vi "002 DataSaveThread.vi"(8 "Caller":refnum<queue>, 9 "Project":string, 10 "Path":path=path "D:/NBT/Code/NBT-TestPlatform 20230715/Config/NBT/NBT_V3.0.0/Default/DataSave/Save/Save01", 11 "Exit":refnum<user-event>) -> ()   [LabVIEW 2020]
uses:
  Alin/QMH/Queue Message.ctl
  9999 SubVI/000_DataSave/Save Type.ctl
  <vilib>/Utility/file.llb/Read Delimited Spreadsheet (string).vi
  <vilib>/Utility/config.llb/Read Key (String).vi
  <vilib>/Utility/config.llb/NI_LVConfig.lvlib
panel:
  out "Wave":waveform(sgl)(graph)
  out "C1":u64(graph)
  out "C2":T1(graph)
  out "C3":i32(graph)
  out "QS":string
  out "QN":i32
  in  "Stop":bool
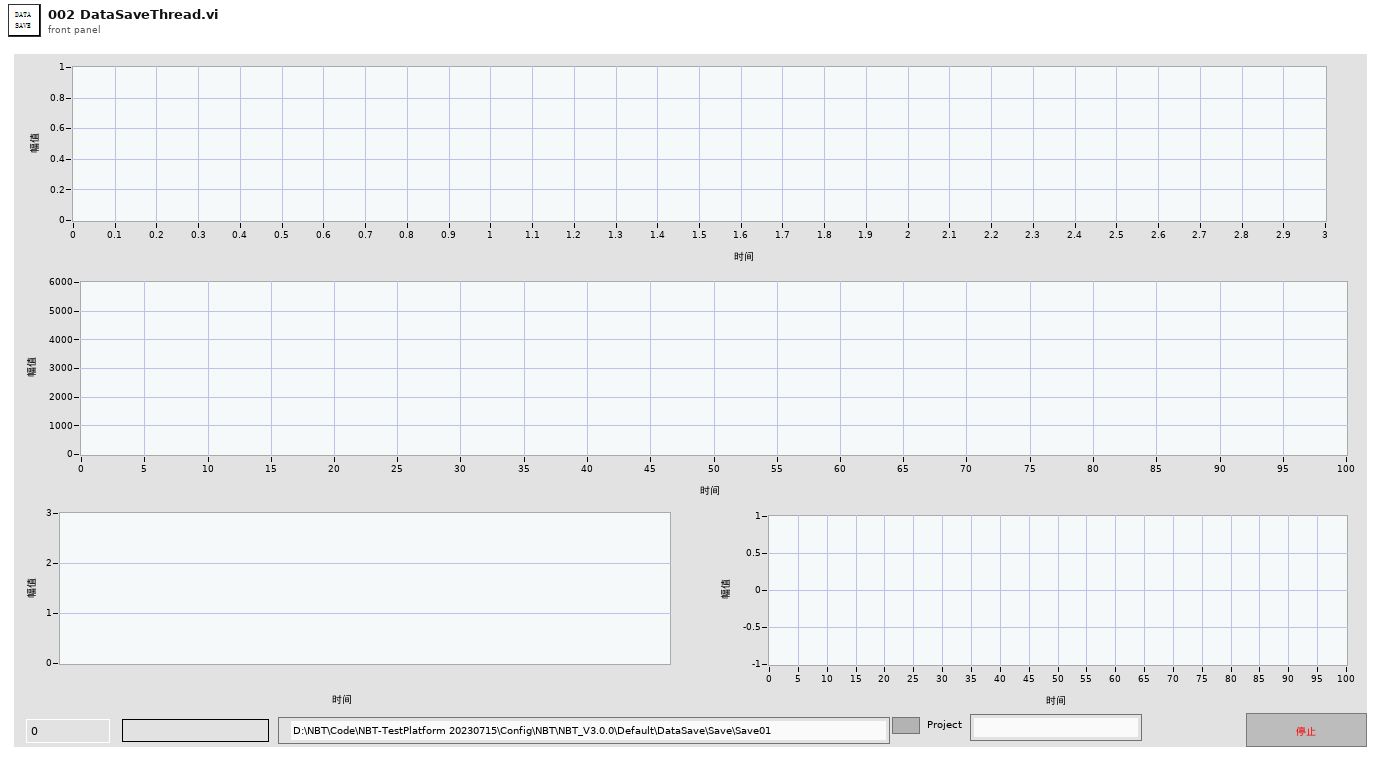
[diagram p1: front panel]
types:
  T1 = cluster{"seconds since 1Jan1904":timestamp, i32}[]
  T2 = typedef "Save Type.ctl" = cluster{"Project":string, "Path":path, "Name":string, "Wave":waveform(sgl)}
  T3 = cluster{"DPath":path, "Last":u64, "Interval":u64, "Max":i32, "File":cluster{"File":string, "Max":i64}, "Wave":map{string, waveform(sgl)}, "Names":string[], "Time":cluster{"UP":u64, "LOW":u64}, "Project":string, "WQ":refnum<queue>, "SQ":map{string, refnum<queue>}, "Save Name":string, "Type":T2, "Caller":refnum<queue>}
  T4 = enum8{"Enabled", "Disabled", "Disabled and Grayed Out"}
  T5 = typedef "NI_LVConfig.lvlib/Config Data RefNum.ctl" = refnum<k1>
  T6 = enum32{"Invalid", "Standard", "Closed", "Hidden", "Minimized", "Maximized"}
  T7 = typedef "SDQ Data Type.ctl" = cluster{"CAN Length":string, "CAN Name":string, "CAN ID":string, "CAN Type":string, "Test Item":string, "Byte Order":string, "Instruction":string, "Control Type":string, "Group":string, "Offset":dbl, "Coefficient":dbl, "Write Enable":bool, "Lable Type":string, "Key?":string, "Set Value":string, "Upper":dbl, "Lower":dbl, "Unit":string, "Formula":string, "Test Item Type":string, "Length":i32, "Address":string, "Name":string, "Identifier":string, "Data Type":string, "Enumerate?":string, "Enumerate List":string, "Data":string, "Source":string}
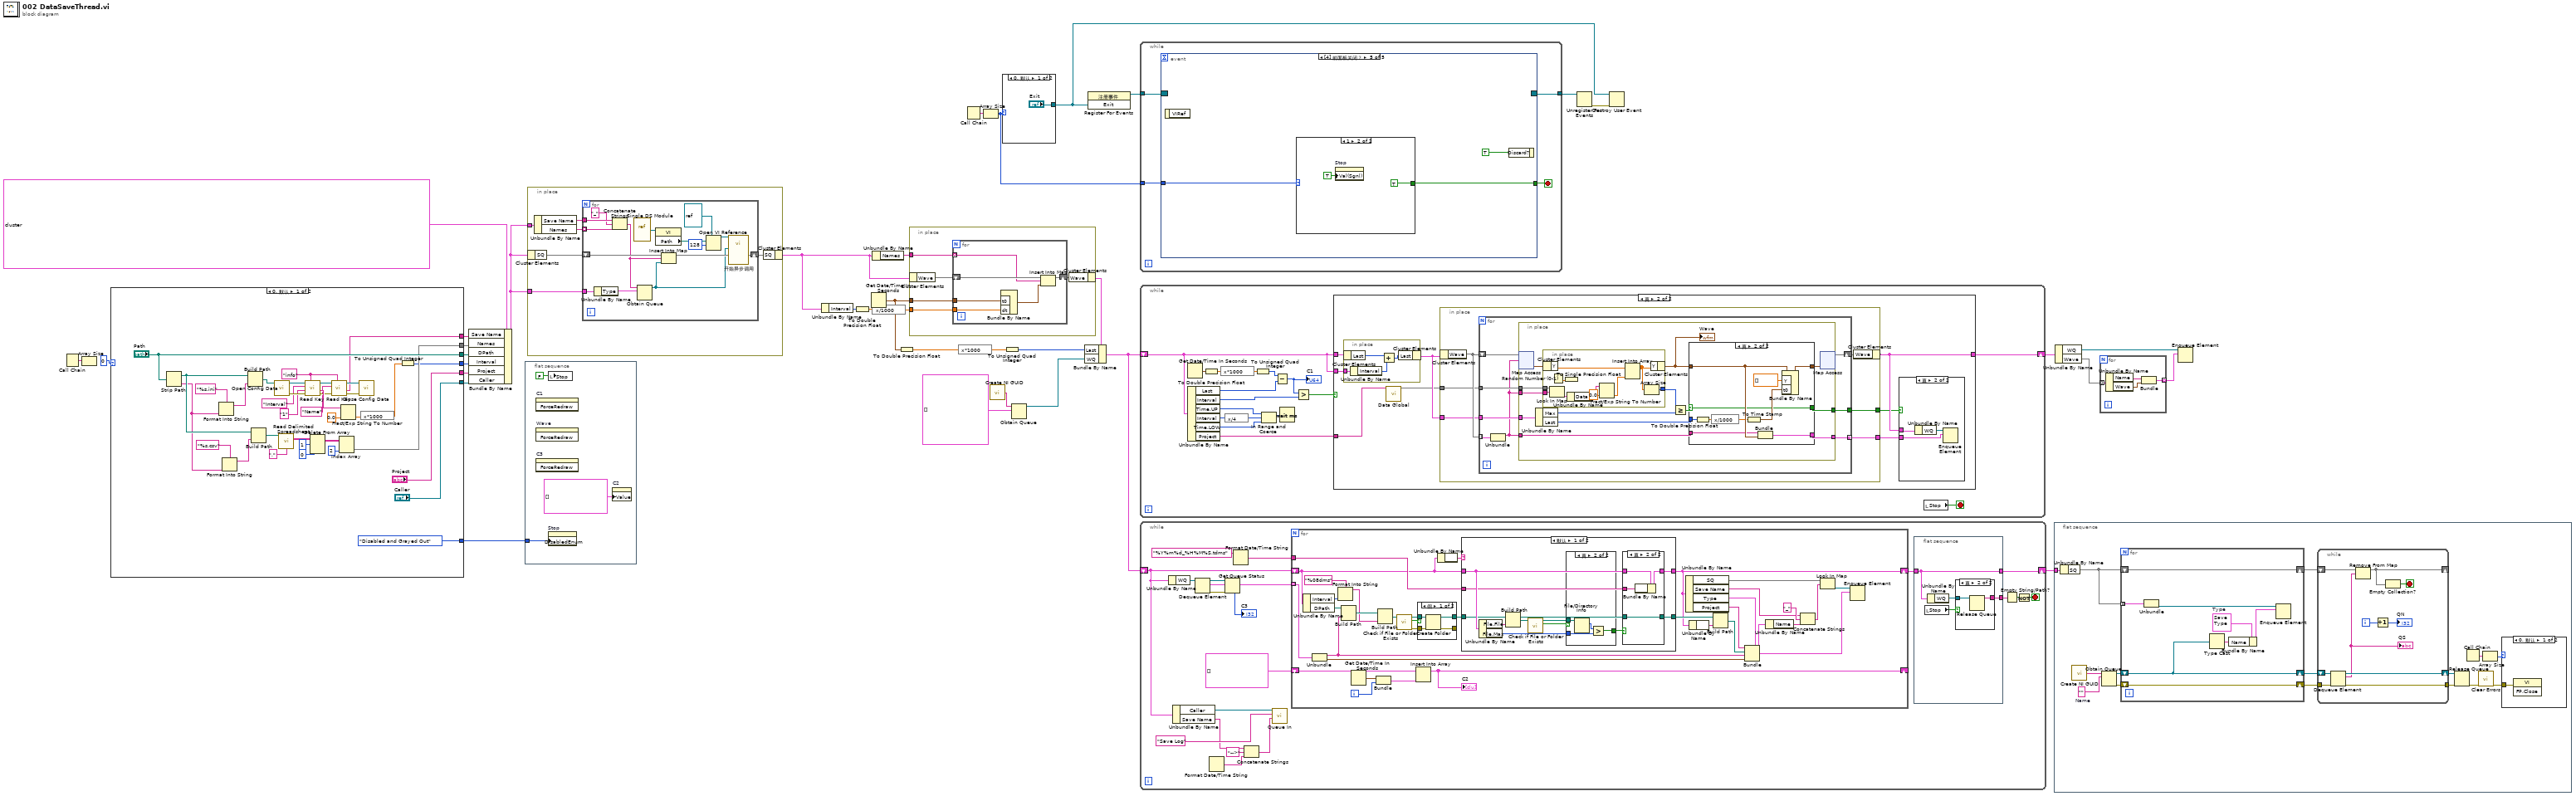
[diagram p0: block diagram]
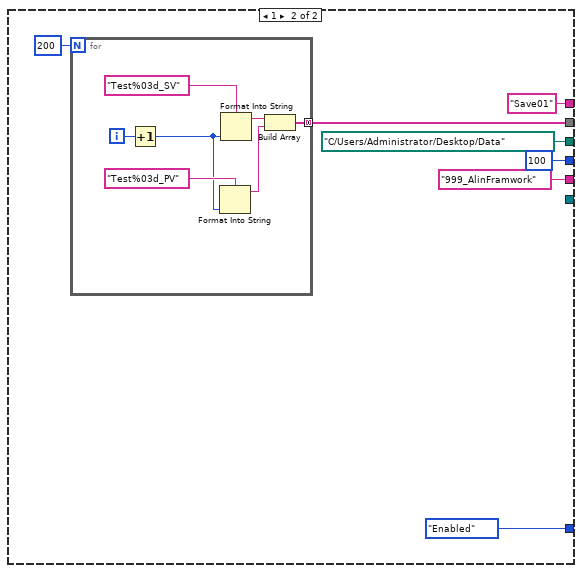
[diagram p2: hidden frame]
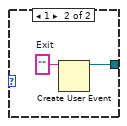
[diagram p3: hidden frame]
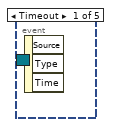
[diagram p5: hidden frame]
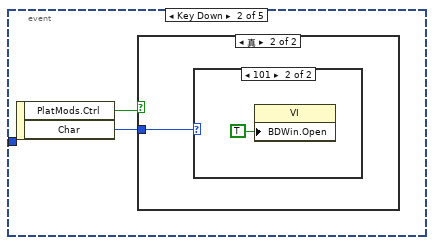
[diagram p6: hidden frame]
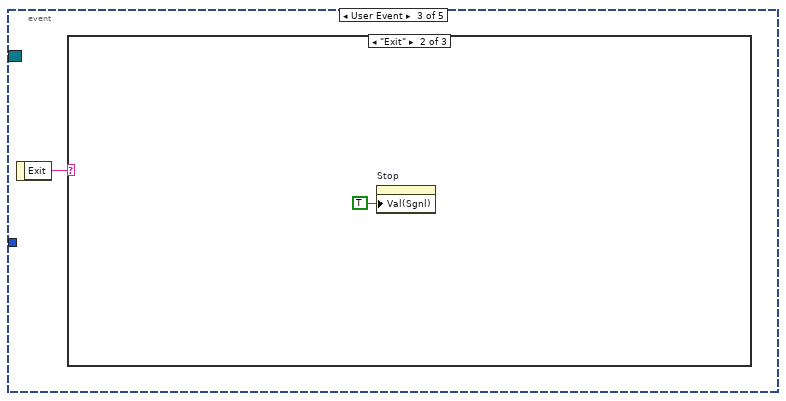
[diagram p9: hidden frame]
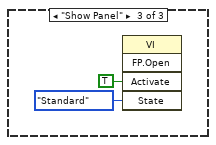
[diagram p11: hidden frame]
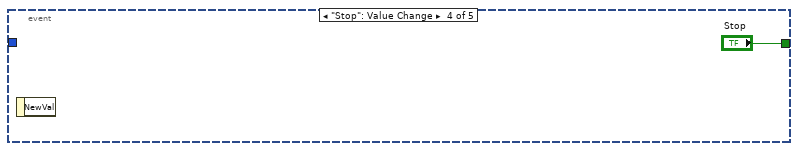
[diagram p12: hidden frame]
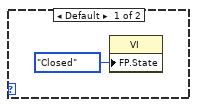
[diagram p13: hidden frame]
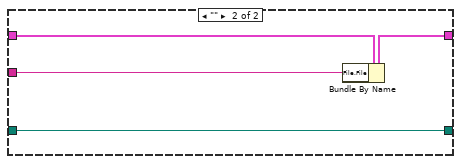
[diagram p17: hidden frame]
diagram:
  n1 = Call Chain() -> (call chain=w11:string[])
  n2 = Array Size(array=w11) -> ()  [unwired: 1 out]
  n3 = case shown="0, 默认" 0 {
    tunnel: ["Path" path "C:/Users/Administrator/Desktop/Data" ("基路径")] -> w26
    tunnel: [w48 u64 100 ("Interval")] -> w25
    tunnel: [w57 w75] -> w23
    tunnel: [T4."Disabled and Grayed Out" ("禁用") T4."Enabled" ("禁用")] -> w9
    tunnel: ["Project" "999_AlinFramwork" ("Project")] -> w8
    tunnel: ["Caller" _] -> w3
    tunnel: [w37 "Save01" ("value")] -> w2
    frame 0, Default {
      w39 = "info" ("section")
      n4 = Strip Path(path="Path") -> (stripped path=w66:path, name=w65:string)
      n5 = Format Into String(format string="%s.ini" ("格式字符串"), w65) -> (resulting string=w69:string)  [unwired: 2 in, 1 out]
      n6 = Format Into String(format string="%s.csv" ("格式字符串"), w65) -> (resulting string=w68:string)  [unwired: 2 in, 1 out]
      n7 = Build Path(base path=w66, name or relative path=w69) -> (appended path=w53:path)
      n8 = Build Path(base path=w66, name or relative path=w68) -> (appended path=w64:path)
      n9 = call <vilib>:"Open Config Data.vi"("configuration file path"=w53) -> ("error out"=w55:errorcluster, "refnum"=w56:T5)  [unwired: 8 in, 1 out]
      n10 = call-poly <vilib>:"Read Delimited Spreadsheet.vi"("file path (dialog if empty)"=w64, "delimiter (\\t)"="," ("delimiter (\\t)")) -> ("all rows"=w62:string[][])  [unwired: 8 in, 5 out]
      n11 = call-poly <vilib>:"Read Key.vi"("section"=w39, "error in (no error)"=w55, "default value"="1", "key"="Interval", "refnum"=w56) -> ("error out"=w42:errorcluster, "value"=w51:string, "refnum out"=w43:T5)  [unwired: 3 in, 1 out]
      n12 = Delete From Array(array=w62, length=1 ("长度"), index (row)=0 ("索引 (行)")) -> (array with subset deleted=w59:string[][])  [unwired: 1 in, 1 out]
      n13 = call-poly <vilib>:"Read Key.vi"("section"=w39, "error in (no error)"=w42, "key"="Name", "refnum"=w43) -> ("error out"=w41:errorcluster, "value"=w37:string, "refnum out"=w40:T5)  [unwired: 4 in, 1 out]
      n14 = Index Array(array=w59, index (col)=2 ("禁用的索引 (列)")) -> (element=w57:string[])  [unwired: 1 in]
      n15 = Fract/Exp String To Number(string=w51, default (0 dbl)=sgl 0.0 ("默认(0 DBL)")) -> (number=w49:sgl)  [unwired: 2 in, 1 out]
      n16 = call <vilib>:"Close Config Data.vi"("error in (no error)"=w41, "refnum"=w40) -> ()  [unwired: 8 in, 2 out]
      n17 = expression code="x*1000"(w49) -> (w47:sgl)
      n18 = To Unsigned Quad Integer(1:w47) -> (0:w48:u64)
    }
    frame 1 {
      n19 = for {
        N: 200 -> [_]
        tunnel: [w80] -> w75 mode=concatenating
        i -> [w83]
        n20 = Increment(x=w83) -> (x+1=w79:i32)
        n21 = Format Into String(format string="Test%03d_PV" ("格式字符串"), w79) -> (resulting string=w81:string)  [unwired: 2 in, 1 out]
        n22 = Format Into String(format string="Test%03d_SV" ("格式字符串"), w79) -> (resulting string=w82:string)  [unwired: 2 in, 1 out]
        n23 = Build Array(w82, w81) -> (w80:string[])
      }
    }
  }
  n24 = Bundle By Name(cluster=T3 {"DPath"=path "", "Last"=0, "Interval"=100, "Max"=100, "File"={"File"="", "Max"=102400}, "Wave"={}, "Names"=[], "Time"={"UP"=500, "LOW"=20}, "Project"="", "WQ"=refnum, "SQ"={}, "Save Name"="Save01", "Type"={"Project"="", "Path"=path "", "Name"="", "Wave"={"t0"=timestamp(0 s since 1904-01-01), "dt"=1.0, "Y"=[]}}, "Caller"=refnum}, "Save Name"=w2, "Names"=w23, "DPath"=w26, "Interval"=w25, "Project"=w8, "Caller"=w3) -> (w18:T3)
  n25 = flat-sequence {
    tunnel: w9 -> [w86]
    frame #0 {
      n26 = invoke on="C1" class="WFChart (严格)" method="ForceRedraw"() -> ()  [unwired: 3 in, 3 out]
      n27 = invoke on="Wave" class="WFGraph (严格)" method="ForceRedraw"() -> ()  [unwired: 3 in, 3 out]
      n28 = invoke on="C3" class="WFChart (严格)" method="ForceRedraw"() -> ()  [unwired: 3 in, 3 out]
      n29 = property on="Stop" class="Bool (严格)"("DisabledEnum"=w86) -> ()  [unwired: 2 in, 2 out]
      n30 = local write "Stop"(FALSE ("Stop")) -> ()
      n31 = property on="C2" class="XYGraph (严格)"("Value"=T1 [] ("C2")) -> ()  [unwired: 2 in, 2 out]
    }
  }
  n32 = in-place {
    in-place-border: w18 -> [w94]
    in-place-border: w18 -> [w89]
    n33 = in-place-cluster #1(w18) -> ("SQ"=w92:map{string, refnum<queue>})
    n34 = Unbundle By Name(w94) -> ("Save Name"=w90:string, "Names"=w93:string[])
    n35 = for {
      tunnel: w93 -> [w106] mode=indexing
      shift-right: [w101] -> w91
      shift-left: w92 -> [w105]
      tunnel: w90 -> [w108]
      tunnel: w89 -> [w103]
      n36 = Unbundle By Name(w103) -> ("Type"=w102:T2)
      n37 = Concatenate Strings(w108, "_" ("字符串"), w106) -> (w104:string)
      n38 = vi-ref "Single DS Module.vi"() -> (w100:refnum<vi>)
      n39 = Obtain Queue(name (unnamed)=w104, element data type=w102) -> (queue out=w95:refnum<queue>)  [unwired: 3 in, 2 out]
      n40 = property class="VI"(reference=w100) -> ("Path"=w99:path)  [unwired: 1 in, 2 out]
      n41 = Insert Into Map(map in=w105, key=w104, value=w95) -> (map out=w101:map{string, refnum<queue>})  [unwired: 2 out]
      n42 = Open VI Reference(type specifier VI Refnum (for type only)=refnum<vi> refnum ("类型说明符VI引用句柄（仅用于类型）"), vi path=w99, options=128 ("选项")) -> (vi reference=w98:refnum<vi>)  [unwired: 3 in, 1 out]
      n43 = call-by-ref "开始异步调用"(reference=w98, "Queue"=w95) -> ()  [unwired: 11 in, 3 out]
    }
    n44 = in-place-cluster #1("SQ"=w91) -> (w7:T3)
  }
  n45 = Unbundle By Name(w7) -> ("Interval"=w6:u64)
  n46 = To Double Precision Float(number=w6) -> (double precision float=w5:dbl)
  n47 = Get Date/Time In Seconds() -> (seconds since 1Jan1904=w33:timestamp)
  n48 = Unbundle By Name(w7) -> ("Names"=w29:string[])
  n49 = expression code="x/1000"(w5) -> (w4:dbl)
  n50 = To Double Precision Float(number=w33) -> (double precision float=w35:dbl)
  n51 = in-place {
    in-place-border: w33 -> [w113]
    in-place-border: w29 -> [w112]
    in-place-border: w4 -> [w109]
    n52 = in-place-cluster #2(w7) -> ("Wave"=w111:map{string, waveform(sgl)})
    n53 = for {
      tunnel: w113 -> [w119]
      tunnel: w109 -> [w118]
      tunnel: w112 -> [w114] mode=indexing
      shift-right: [w116] -> w110
      shift-left: w111 -> [w117]
      n54 = Bundle By Name("t0"=w119, "dt"=w118) -> (w115:waveform(dbl))  [unwired: 1 in]
      n55 = Insert Into Map(map in=w117, key=w114, value=w115) -> (map out=w116:map{string, waveform(sgl)})  [unwired: 2 out]
    }
    n56 = in-place-cluster #2("Wave"=w110) -> (w36:T3)
  }
  n57 = expression code="x*1000"(w35) -> (w34:dbl)
  n58 = Call Chain() -> (call chain=w12:string[])
  n59 = Array Size(array=w12) -> (size(s)=w1:i32)
  n60 = call <vilib>:"Create NI GUID.vi"() -> ("NI GUID"=w27:string)
  n61 = case shown="0, 默认" w1 {
    tunnel: ["Exit" w121] -> w13
    frame 0, Default {
    }
    frame 1 {
      w122 = ""  # Exit
      n62 = Create User Event(user event datatype=w122) -> (user event=w121:refnum<user-event>)  [unwired: 1 in, 1 out]
    }
  }
  n63 = To Unsigned Quad Integer(1:w34) -> (0:w32:u64)
  n64 = Obtain Queue(name (unnamed)=w27, element data type=cluster{"Name":string, "Wave":waveform(sgl)}[] [] ("输出簇")) -> (queue out=w24:refnum<queue>)  [unwired: 3 in, 2 out]
  n65 = Bundle By Name(cluster=w36, "Last"=w32, "WQ"=w24) -> (w31:T3)
  n66 = register-events(w13) -> (reference out=w16:refnum<event-registration>)  [unwired: 2 in, 1 out]
  n67 = while {
    tunnel: w16 -> [w125]
    tunnel: [w124] -> w15
    tunnel: w1 -> [w123]
    stop <- w126 stop-if-true
    n68 = event shown="[4] 前面板关闭？" {
      selector: w125 -> [_ _ _ _ _]
      dyn-events: [_ _ _ _ _] -> w124
      timeout: _ -> [_ _ _ _ _]
      tunnel: [_ _ _ "Stop" w136] -> w126
      tunnel: w123 -> [_ _ _ _ w137]
      event Timeout {
        n69 = event-data() -> ()  [unwired: 1 in, 3 out]
      }
      event Key Down {
        n70 = event-data() -> ("PlatMods.Ctrl"=w128:bool, "Char"=w127:i16)  [unwired: 1 in]
        n71 = case shown="真" w128 {
          tunnel: w127 -> [_ w129]
          frame False {
          }
          frame True {
            n72 = case shown="101" w129 {
              frame 0, Default {
              }
              frame 101 {
                n73 = property class="VI"("BDWin.Open"=TRUE ("程序框图窗口:打开")) -> ()  [unwired: 2 in, 2 out]
              }
            }
          }
        }
      }
      event User Event {
        n74 = event-data() -> ("Exit"=w131:string)  [unwired: 1 in]
        n75 = case shown="\"Exit\"" w131 {
          frame "假", Default {
          }
          frame "Exit" {
            n76 = property on="Stop" class="Bool (严格)"("Val(Sgnl)"=TRUE ("值(信号)")) -> ()  [unwired: 2 in, 2 out]
          }
          frame "Show Panel" {
            n77 = invoke class="VI" method="FP.Open"("Activate"=TRUE ("激活？"), "State"=T6."Standard" ("状态")) -> ()  [unwired: 3 in, 5 out]
          }
        }
      }
      event "Stop": Value Change {
        n78 = event-data() -> ()  [unwired: 1 in, 1 out]
      }
      event Panel Close? {
        n79 = event-data() -> ()  [unwired: 1 in, 1 out]
        n80 = case shown="1" w137 {
          tunnel: [_ TRUE] -> w136
          frame Default {
            n81 = property class="VI"("FP.State"=T6."Closed" ("前面板窗口:状态")) -> ()  [unwired: 2 in, 2 out]
          }
          frame 1 {
            n82 = property on="Stop" class="Bool (严格)"("Val(Sgnl)"=TRUE ("值(信号)")) -> ()  [unwired: 2 in, 2 out]
          }
        }
        n83 = event-data("Discard?"=TRUE ("放弃？")) -> ()  [unwired: 1 in, 1 out]
      }
    }
  }
  n84 = while {
    shift-right: [w153] -> w21
    shift-left: w31 -> [w143]
    stop <- w144 stop-if-true
    n85 = Get Date/Time In Seconds() -> (seconds since 1Jan1904=w158:timestamp)
    n86 = Unbundle By Name(w143) -> ("Last"=w152:u64, "Interval"=w150:u64, "Time.UP"=w147:u64, "Interval"=w146:u64, "Time.LOW"=w145:u64, "Project"=w142:string)
    n87 = To Double Precision Float(number=w158) -> (double precision float=w157:dbl)
    n88 = expression code="x*1000"(w157) -> (w156:dbl)
    n89 = expression code="x/4"(w146) -> (w149:u64)
    n90 = To Unsigned Quad Integer(1:w156) -> (0:w155:u64)
    n91 = In Range and Coerce(upper limit=w147, x=w149, lower limit=w145) -> (coerced(x)=w148:u64)  [unwired: 1 out]
    n92 = Subtract(x=w155, y=w152) -> (x-y=w151:u64)
    "C1" <- w151
    n93 = Wait (ms)(milliseconds to wait=w148) -> ()  [unwired: 1 out]
    n94 = Greater?(x=w151, y=w150) -> (0:w154:bool)
    n95 = case shown="真" w154 {
      tunnel: w143 -> [w159 w167]
      tunnel: [w159 w165] -> w153
      tunnel: w143 -> [_ w162]
      tunnel: w142 -> [_ w161]
      frame False {
      }
      frame True {
        n96 = in-place {
          in-place-border: w162 -> [w173]
          n97 = in-place-cluster #3(w167) -> ("Last"=w174:u64)
          n98 = Unbundle By Name(w173) -> ("Interval"=w172:u64)
          n99 = Add(x=w174, y=w172) -> (x+y=w171:u64)
          n100 = in-place-cluster #3("Last"=w171) -> (w166:T3)
        }
        n101 = call "Data Global.vi"("Name"=w161) -> ("Data Out"=w160:map{string, T7})  [unwired: 7 in, 3 out]
        n102 = in-place {
          in-place-border: w166 -> [w178]
          in-place-border: [w177] -> w164
          in-place-border: [w176] -> w163
          in-place-border: w160 -> [w175]
          n103 = in-place-cluster #4(w166) -> ("Wave"=w180:map{string, waveform(sgl)})
          n104 = for {
            tunnel: w180 -> [w188] mode=indexing
            shift-right: [w186] -> w179
            shift-left: w180 -> [w187]
            tunnel: w178 -> [w185]
            tunnel: [w184] -> w177 mode=indexing
            tunnel: [w183] -> w176
            tunnel: w175 -> [w182]
            n105 = Unbundle(w188) -> ("Name"=w181:string)  [unwired: 1 out]
            n106 = in-place {
              in-place-border: w181 -> [w196]
              in-place-border: w185 -> [w193]
              in-place-border: [w192] -> w184
              in-place-border: [w191] -> w183
              in-place-border: w182 -> [w190]
              in-place-border: w181 -> [w189]
              n107 = in-place-map #5(w187, w181) -> (w197:waveform(sgl))  [unwired: 1 in, 1 out]
              n108 = Unbundle By Name(w193) -> ("Max"=w200:i32, "Last"=w194:u64)
              n109 = in-place {
                in-place-border: [w221] -> w201
                in-place-border: w190 -> [w218]
                in-place-border: w189 -> [w213]
                n110 = in-place-cluster #6(w197) -> ("Y"=w222:sgl[])
                n111 = Look In Map(map=w218, key=w213) -> (value=w217:T7)  [unwired: 1 in, 1 out]
                n112 = Random Number (0-1)() -> (number: 0 to 1=w219:dbl)
                n113 = To Single Precision Float(number=w219) -> ()  [unwired: 1 out]
                n114 = Unbundle By Name(w217) -> ("Data"=w216:string)
                n115 = Fract/Exp String To Number(string=w216, default (0 dbl)=sgl 0.0 ("默认(0 DBL)")) -> (number=w215:sgl)  [unwired: 2 in, 1 out]
                n116 = Insert Into Array(array=w222, new element=w215) -> (w220:sgl[])  [unwired: 1 in]
                n117 = Array Size(array=w220) -> (size(s)=w221:i32)
                n118 = in-place-cluster #6("Y"=w220) -> (w198:waveform(sgl))
              }
              "Wave" <- w198
              n119 = Greater Or Equal?(x=w201, y=w200) -> (x >= y?=w199:bool)
              n120 = case shown="真" w199 {
                selector: w199 -> [_ w203]
                tunnel: w198 -> [w202 w210]
                tunnel: [w202 w211] -> w195
                tunnel: w194 -> [_ w209]
                tunnel: w196 -> [_ w205]
                tunnel: [_ w204] -> w192
                tunnel: [_ w203] -> w191
                frame False {
                }
                frame True {
                  n121 = To Double Precision Float(number=w209) -> (double precision float=w208:dbl)
                  n122 = expression code="x/1000"(w208) -> (w207:dbl)
                  n123 = To Time Stamp(1:w207) -> (0:w206:timestamp)
                  n124 = Bundle("Name"=w205, "Wave"=w210) -> (w204:cluster{"Name":string, "Wave":waveform(sgl)})  [unwired: 1 in]
                  n125 = Bundle By Name(cluster=w210, "Y"=sgl[] [], "t0"=w206) -> (w211:waveform(sgl))
                }
              }
              n126 = in-place-map #5(w195) -> (w186:map{string, waveform(sgl)})  [unwired: 1 in, 2 out]
            }
          }
          n127 = in-place-cluster #4("Wave"=w179) -> (w165:T3)
        }
        n128 = case shown="真" w163 {
          tunnel: w165 -> [_ w170]
          tunnel: w164 -> [_ w168]
          frame False {
          }
          frame True {
            n129 = Unbundle By Name(w170) -> ("WQ"=w169:refnum<queue>)
            n130 = Enqueue Element(queue=w169, element=w168) -> ()  [unwired: 2 in, 3 out]
          }
        }
      }
    }
    n131 = local read "Stop"() -> (w144:bool)
  }
  n132 = while {
    shift-right: [w234] -> w17
    shift-left: w31 -> [w229]
    stop <- w237 stop-if-true
    n133 = Unbundle By Name(w229) -> ("WQ"=w241:refnum<queue>)
    n134 = Unbundle By Name(w229) -> ("Caller"=w228:refnum<queue>, "Save Name"=w226:string)
    n135 = Dequeue Element(queue=w241) -> (queue out=w232:refnum<queue>, element=w242:cluster{"Name":string, "Wave":waveform(sgl)}[], error out=w231:errorcluster)  [unwired: 2 in, 1 out]
    n136 = Format Date/Time String() -> (date/time string=w224:string)  [unwired: 3 in]
    n137 = Get Queue Status(queue=w232, error in (no error)=w231) -> (# elements in queue=→"C3":i32)  [unwired: 1 in, 7 out]
    n138 = Format Date/Time String(time format string (%c)="%Y%m%d_%H%M%S.tdms" ("时间格式字符串(%c)")) -> (date/time string=w239:string)  [unwired: 2 in]
    n139 = Concatenate Strings(w226, "-->" ("字符串"), w224) -> (w223:string)
    n140 = call "Queue In.vi"("Data"=w223, "Message"="Save Log", "Queue In"=w228) -> ()  [unwired: 7 in, 2 out]
    n141 = for {
      tunnel: w242 -> [w282] mode=indexing
      shift-right: [w269] -> w235
      shift-left: w229 -> [w251]
      tunnel: w239 -> [w270]
      shift-right: [w260] -> _
      shift-left: T1 [] ("输出簇") -> [w262]
      i -> [w263]
      n142 = Unbundle By Name(w251) -> ("Interval"=w250:u64, "DPath"=w249:path)
      n143 = Unbundle(w282) -> ("Name"=w266:string, "Wave"=w265:waveform(sgl))
      n144 = Format Into String(format string="%08dms" ("格式字符串"), w250) -> (resulting string=w275:string)  [unwired: 2 in, 1 out]
      n145 = Build Path(base path=w249, name or relative path=w266) -> (appended path=w277:path)
      n146 = Get Date/Time In Seconds() -> (seconds since 1Jan1904=w264:timestamp)
      n147 = Bundle("seconds since 1Jan1904"=w264, w263) -> (w261:cluster{"seconds since 1Jan1904":timestamp, i32})  [unwired: 1 in]
      n148 = Build Path(base path=w277, name or relative path=w275) -> (appended path=w276:path)
      n149 = call <vilib>:"Check if File or Folder Exists.vi"("path"=w276) -> ("error out"=w281:errorcluster, "file or folder exists?"=w279:bool, "dup path"=w280:path)  [unwired: 8 in]
      n150 = Insert Into Array(array=w262, new element=w261) -> (w260:T1)  [unwired: 1 in]
      "C2" <- w260
      n151 = case shown="假" w279 {
        tunnel: w280 -> [w311 w313]
        tunnel: w281 -> [w310 w312]
        tunnel: [w309 w313] -> w273
        tunnel: [w308 w312] -> _
        frame False {
          n152 = Create Folder(path (use dialog)=w311, error in=w310) -> (created path=w309:path, error out=w308:errorcluster)  [unwired: 1 in, 1 out]
        }
        frame True {
        }
      }
      n153 = Unbundle By Name(w251) -> ("File.File"=w274:string)
      n154 = case shown="默认" w274 {
        tunnel: w270 -> [w284 w306]
        tunnel: w273 -> [w288 w304]
        tunnel: w251 -> [w290 w307]
        tunnel: [w289 w305] -> w269
        tunnel: [w287 w304] -> w272
        frame Default {
          n155 = Unbundle By Name(w290) -> ("File.File"=w293:string, "File.Max"=w292:i64)
          n156 = Build Path(base path=w288, name or relative path=w293) -> (appended path=w286:path)
          n157 = call <vilib>:"Check if File or Folder Exists.vi"("path"=w286) -> ("file or folder exists?"=w283:bool, "dup path"=w285:path)  [unwired: 8 in, 1 out]
          n158 = case shown="真" w283 {
            tunnel: w292 -> [_ w296]
            tunnel: [_ w295] -> w291
            tunnel: w285 -> [_ w294]
            frame False {
            }
            frame True {
              n159 = File/Directory Info(path=w294) -> (size=w297:i64)  [unwired: 1 in, 6 out]
              n160 = Greater?(x=w297, y=w296) -> (0:w295:bool)
            }
          }
          n161 = case shown="真" w291 {
            tunnel: w284 -> [_ w301]
            tunnel: w290 -> [w299 w303]
            tunnel: [w299 w302] -> w289
            tunnel: w288 -> [w298 w300]
            tunnel: [w298 w300] -> w287
            frame False {
            }
            frame True {
              n162 = Bundle By Name(cluster=w303, "File.File"=w301) -> (w302:T3)
            }
          }
        }
        frame "" {
          n163 = Bundle By Name(cluster=w307, "File.File"=w306) -> (w305:T3)
        }
      }
      n164 = Unbundle By Name(w269) -> ("SQ"=w255:map{string, refnum<queue>}, "Save Name"=w257:string, "Type"=w259:T2, "Project"=w268:string)
      n165 = Unbundle By Name(w269) -> ("File.File"=w271:string)
      n166 = Build Path(base path=w272, name or relative path=w271) -> (appended path=w267:path)
      n167 = Bundle(cluster=w259, "Project"=w268, "Path"=w267, "Name"=w266, "Wave"=w265) -> (w252:T2)
      n168 = Unbundle By Name(w252) -> ("Name"=w256:string)
      n169 = Concatenate Strings(w257, "_" ("字符串"), w256) -> (w254:string)
      n170 = Look In Map(map=w255, key=w254) -> (value=w253:refnum<queue>)  [unwired: 1 in, 1 out]
      n171 = Enqueue Element(queue=w253, element=w252) -> ()  [unwired: 2 in, 3 out]
    }
    n172 = flat-sequence {
      tunnel: [w245] -> w238
      tunnel: w235 -> [w243]
      tunnel: [w243] -> w234
      frame #0 {
        n173 = local read "Stop"() -> (w246:bool)
        n174 = Unbundle By Name(w243) -> ("WQ"=w244:refnum<queue>)
        n175 = case shown="真" w246 {
          tunnel: w244 -> [_ w248]
          tunnel: [_ w247] -> w245
          frame False {
          }
          frame True {
            n176 = Release Queue(queue=w248) -> (queue name=w247:string)  [unwired: 2 in, 2 out]
          }
        }
      }
    }
    n177 = Empty String/Path?(string/path=w238) -> (empty?=w236:bool)
    n178 = Not(x=w236) -> (.not. x?=w237:bool)
  }
  n179 = Unregister For Events(event registration refnum=w15) -> (error out=w14:errorcluster)  [unwired: 1 in]
  n180 = Destroy User Event(user event=w13, error in=w14) -> ()  [unwired: 1 out]
  n181 = flat-sequence {
    tunnel: w17 -> [w328]
    frame #0 {
      w326 = ""  # Name
      n182 = Unbundle By Name(w328) -> ("SQ"=w324:map{string, refnum<queue>})
      n183 = call <vilib>:"Create NI GUID.vi"() -> ("NI GUID"=w327:string)
      n184 = Obtain Queue(name (unnamed)=w327, element data type=w326) -> (queue out=w325:refnum<queue>, error out=w319:errorcluster)  [unwired: 3 in, 1 out]
      n185 = for {
        tunnel: w324 -> [w347] mode=indexing
        shift-right: [w342] -> w322
        shift-left: w325 -> [w342]
        shift-right: [w341] -> w323
        shift-left: w324 -> [w341]
        shift-right: [w340] -> w318
        shift-left: w319 -> [w340]
        w345 = T2 {"Project"="Exit", "Path"=path "", "Name"="", "Wave"={"t0"=timestamp(0 s since 1904-01-01), "dt"=1.0, "Y"=[]}}  # Type
        n186 = Unbundle(w347) -> ("DQ"=w346:refnum<queue>)  [unwired: 1 out]
        n187 = Type Cast(x=w342) -> (*(type *) &x=w343:string)  [unwired: 1 in]
        n188 = Bundle By Name(cluster=w345, "Name"=w343) -> (w344:T2)
        n189 = Enqueue Element(queue=w346, element=w344) -> ()  [unwired: 2 in, 3 out]
      }
      n190 = while {
        shift-right: [w337] -> _
        shift-left: w323 -> [w338]
        shift-right: [w335] -> w321
        shift-left: w322 -> [w339]
        tunnel: [w334] -> w320
        tunnel: w318 -> [w333]
        i -> [w332]
        stop <- w336 stop-if-true
        n191 = Dequeue Element(queue=w339, error in (no error)=w333) -> (queue out=w335:refnum<queue>, element=w331:string, error out=w334:errorcluster)  [unwired: 1 in, 1 out]
        "QS" <- w331
        n192 = Remove From Map(10:w331, 11:w338) -> (3:w337:map{string, refnum<queue>})  [unwired: 2 out]
        n193 = Increment(x=w332) -> (x+1=→"QN":i32)
        n194 = Empty Collection?(1:w337) -> (0:w336:bool)
      }
      n195 = Release Queue(queue=w321, error in (no error)=w320) -> (error out=w315:errorcluster)  [unwired: 1 in, 2 out]
      n196 = Call Chain() -> (call chain=w317:string[])
      n197 = call <vilib>:"Clear Errors.vi"("error in (no error)"=w315) -> ("error out"=w314:errorcluster)  [unwired: 5 in, 1 out]
      n198 = Array Size(array=w317) -> (size(s)=w316:i32)
      n199 = case shown="0, 默认" w316 {
        tunnel: w314 -> [w329 _]
        frame 0, Default {
          n200 = invoke class="VI" method="FP.Close"(error in=w329) -> ()  [unwired: 2 in, 3 out]
        }
        frame 1 {
        }
      }
    }
  }
  n201 = Unbundle By Name(w21) -> ("WQ"=w22:refnum<queue>, "Wave"=w20:map{string, waveform(sgl)})
  n202 = for {
    tunnel: w20 -> [w351] mode=indexing
    tunnel: [w348] -> w19 mode=indexing
    n203 = Unbundle By Name(w351) -> ("Name"=w350:string, "Wave"=w349:waveform(sgl))
    n204 = Bundle("Name"=w350, "Wave"=w349) -> (w348:cluster{"Name":string, "Wave":waveform(sgl)})  [unwired: 1 in]
  }
  n205 = Enqueue Element(queue=w22, element=w19) -> ()  [unwired: 2 in, 3 out]
